vi "Create Client.vi"(8 "error in":errorcluster, 11 "cluster id":string) -> (0 "error out":errorcluster, 3 "grpc client id":T1)   [LabVIEW 2021, in "NI Session Management V1 Client.lvlib" / "Session Reservation.lvclass"]
uses:
  Session Reservation.lvclass
  Session Reservation.lvclass/Session Reservation.ctl
  gRPC/Generated APIs/ni/measurementlink/sessionmanagement/v1/ni.measurementlink.sessionmanagement.v1.api.lvlib
  Discovery V1/NI Discovery V1 Client.lvlib
  gRPC/Generated APIs/ni/measurementlink/discovery/v1/RPC Messages/ni_measurementlink_discovery_v1_ResolveServiceRequest.ctl
  gRPC/Generated APIs/ni/measurementlink/discovery/v1/ni.measurementlink.discovery.v1.api.lvlib
  <vilib>/gRPC/LabVIEW gRPC Library/Shared/grpcId.ctl
  <vilib>/gRPC/LabVIEW gRPC Library/grpc-lvsupport-release.lvlib
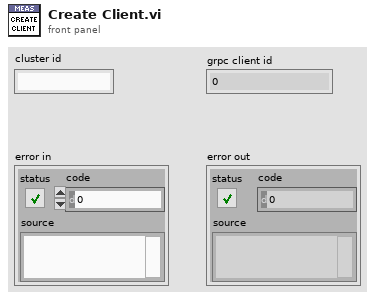
[diagram p1: front panel]
types:
  T1 = typedef "grpc-lvsupport-release.lvlib/grpcId.ctl" = u64
  T2 = typedef "ni.measurementlink.discovery.v1.api.lvlib/ni_measurementlink_discovery_v1_ResolveServiceRequest.ctl" = cluster{"provided_interface":string, "service_class":string, "deployment_target":string, "version":string}
  T3 = typedef "ni.measurementlink.discovery.v1.api.lvlib/ni_measurementlink_discovery_v1_ServiceLocation.ctl" = cluster{"location":string, "insecure_port":string, "ssl_authenticated_port":string}
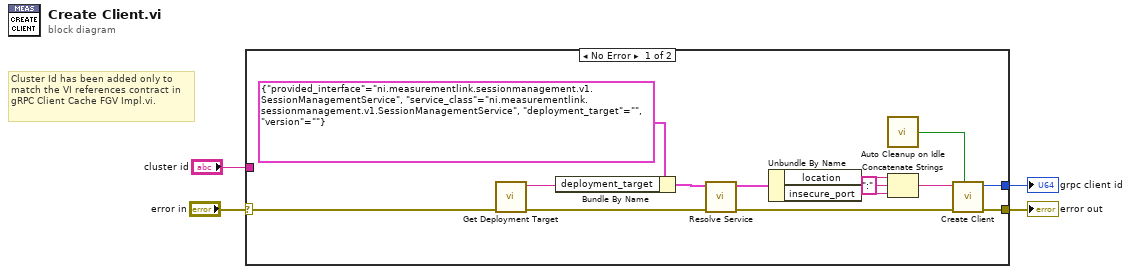
[diagram p0: block diagram]
diagram:
  # "Cluster Id has been added only to match the VI references contract in gRPC Client Cache FGV Impl.vi."
  n1 = case shown="No Error" "error in" {
    selector: "error in" -> [w10 w19]
    tunnel: [w16 _] -> w3
    tunnel: [w15 w19] -> w2
    tunnel: "cluster id" -> [_ _]
    frame No Error {
      n2 = call "Get Deployment Target.vi"("error in (no error)"=w10) -> ("error out"=w9:errorcluster, "deployment target"=w6:string)  [unwired: 9 in]
      n3 = Bundle By Name(cluster=T2 {"provided_interface"="ni.measurementlink.sessionmanagement.v1.SessionManagementService", "service_class"="ni.measurementlink.sessionmanagement.v1.SessionManagementService", "deployment_target"="", "version"=""} ("request data"), "deployment_target"=w6) -> (w7:T2)
      n4 = call "Resolve Service.vi"("error in"=w9, "request data"=w7) -> ("error out"=w17:errorcluster, "response data"=w18:T3)  [unwired: 8 in]
      n5 = Unbundle By Name(w18) -> ("location"=w11:string, "insecure_port"=w12:string)
      n6 = call "Auto Cleanup on Idle.vi"() -> ("auto cleanup"=w5:bool)  [unwired: 1 in]
      n7 = Concatenate Strings(w11, ":" ("string"), w12) -> (w14:string)
      n8 = call "Create Client.vi"("auto cleanup"=w5, "error in"=w17, "address"=w14) -> ("error out"=w15:errorcluster, "gRPC ID Out"=w16:T1)  [unwired: 7 in]
    }
    frame Error {
    }
  }
  "grpc client id" <- w3
  "error out" <- w2
